vi "SpecSave.vi"(10 "Path":path, 11 "Array":dbl[][](array[numeric])) -> ()   [LabVIEW 2013, in "HamamatsuSpectrometerDAQ.lvclass"]
uses:
  HamamatsuSpectrometerDAQ.lvclass
  <vilib>/Utility/file.llb/Write To Spreadsheet File (DBL).vi
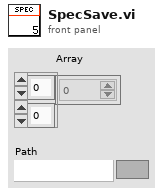
[diagram p1: front panel]
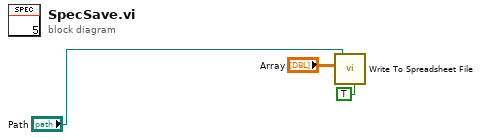
[diagram p0: block diagram]
diagram:
  n1 = call-poly <vilib>:"Write To Spreadsheet File.vi"("transpose? (no:F)"=TRUE, "2D data"="Array", "file path (dialog if empty)"="Path") -> ()  [unwired: 3 in, 3 out]
